vi "Toldo.vi"() -> ()   [LabVIEW 2018]
panel:
  out "Bajar Toldo":bool
  out "Frío":bool
  out "Viento":bool
  out "Lluvia":bool
  out "Sol":bool
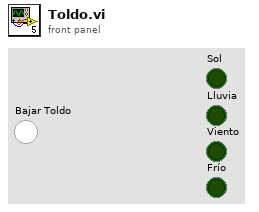
[diagram p1: front panel]
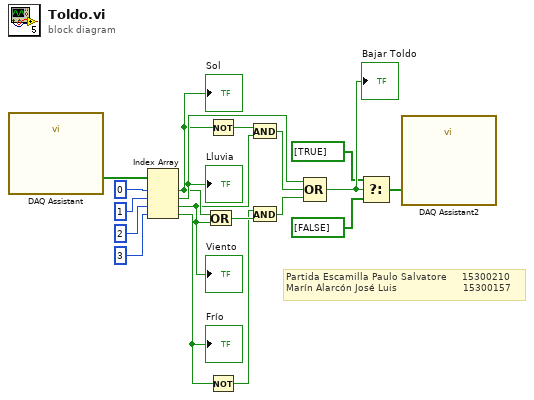
[diagram p0: block diagram]
diagram:
  # "Partida Escamilla Paulo Salvatore     15300210\nMarín Alarcón José Luis                      15300157"
  n1 = call "DAQ Assistant"() -> ("data"=w14:bool[])  [unwired: 17 in, 2 out]
  n2 = Index Array(array=w14, index #1=0 ("index"), index #2=1 ("index"), index #3=2 ("index"), index #4=3 ("index")) -> (element #1=w10:bool, element #2=w13:bool, element #3=w9:bool, element #4=w8:bool)
  "Sol" <- w10
  "Lluvia" <- w13
  "Viento" <- w9
  "Frío" <- w8
  n3 = Or(x=w10, y=w9) -> (x .or. y?=w7:bool)
  n4 = Not(x=w10) -> (.not. x?=w12:bool)
  n5 = Not(x=w8) -> (.not. x?=w6:bool)
  n6 = And(x=w12, y=w9) -> (x .and. y?=w11:bool)
  n7 = And(x=w6, y=w7) -> (x .and. y?=w5:bool)
  n8 = Compound Arithmetic op=OR(w13, w11, w5) -> (w4:bool)
  "Bajar Toldo" <- w4
  n9 = Select(t=bool[] [TRUE] ("data"), s=w4, f=bool[] [FALSE] ("data")) -> (s? t:f=w1:bool[])
  n10 = call "DAQ Assistant2"("data"=w1) -> ()  [unwired: 17 in, 2 out]
